vi "Set Indicators to Default.vi"(4 "error in":errorcluster, 7 "Call Level (2)":i32=2) -> (0 "error out":errorcluster {"code" format="%.0x"})   [LabVIEW 2010]
doc: "This function sets all of the control \"indicators\" on a calling VI front panel to their default values. The input error status does not affect attempting to set the defaults."
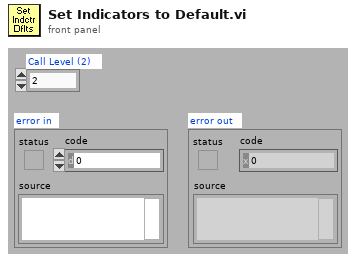
[diagram p1: front panel]
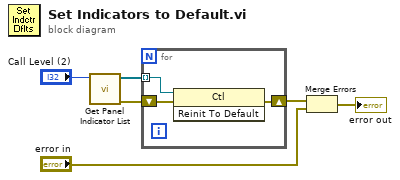
[diagram p0: block diagram]
diagram:
  n1 = call "Get Panel Indicator List.vi"("Call Level (3)"="Call Level (2)") -> ("error out"=w3:errorcluster, "indicator list"=w2:refnum<vi>[])  [unwired: 4 in, 1 out]
  n2 = for {
    shift-right: [w9] -> w4
    shift-left: w3 -> [w8]
    tunnel: w2 -> [w7] mode=indexing
    n3 = invoke class="Ctl" method="Reinit To Default"(reference=w7, error in=w8) -> (error out=w9:errorcluster)  [unwired: 1 in, 2 out]
  }
  n4 = Merge Errors(w4, "error in") -> (→"error out":errorcluster)
